vi "Set Pulse Time to Minimum.vi"(6 "Time":i32(ring)=10214 items=["High"=10192, "Low"=10214], 8 "error in (no error)":errorcluster, 11 "Refnum in":refnum<k21>) -> (0 "error out":errorcluster, 2 "CO.Pulse.Freq":dbl, 3 "Refnum out":refnum<k21>)   [LabVIEW 2015]
uses:
  <resource>/objmgr/daqmx.rc
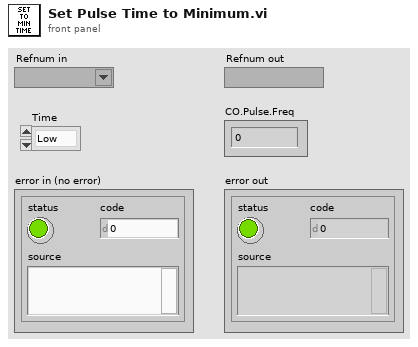
[diagram p1: front panel]
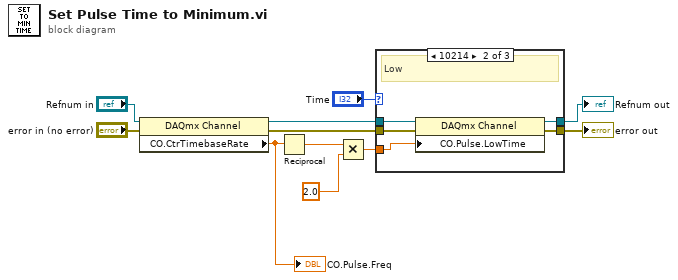
[diagram p0: block diagram]
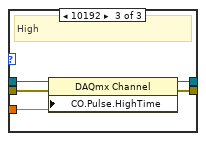
[diagram p3: hidden frame]
diagram:
  n1 = property class="DAQmx Channel"(reference="Refnum in", error in="error in (no error)") -> (reference out=w10:refnum<k21>, error out=w5:errorcluster, "CO.CtrTimebaseRate"=w8:dbl)
  "CO.Pulse.Freq" <- w8
  n2 = Reciprocal(x=w8) -> (1/x=w4:dbl)
  n3 = Multiply(x=w4, y=2.0) -> (x*y=w2:dbl)
  n4 = case shown="10214" "Time" {
    tunnel: w10 -> [w13 w18 w23]
    tunnel: [w13 w15 w22] -> w7
    tunnel: w5 -> [w12 w17 w21]
    tunnel: w2 -> [_ w16 w20]
    tunnel: [w12 w14 w19] -> w1
    frame Default {
    }
    frame 10214 {
      # "Low"
      n5 = property class="DAQmx Channel"(reference=w18, error in=w17, "CO.Pulse.LowTime"=w16) -> (reference out=w15:refnum<k21>, error out=w14:errorcluster)
    }
    frame 10192 {
      # "High"
      n6 = property class="DAQmx Channel"(reference=w23, error in=w21, "CO.Pulse.HighTime"=w20) -> (reference out=w22:refnum<k21>, error out=w19:errorcluster)
    }
  }
  "Refnum out" <- w7
  "error out" <- w1
